vi "Create New File.vi"(8 "error in (no error)":errorcluster, 10 "Path":path, 11 "CSV File in":refnum<class "CSV File.lvclass">) -> (0 "error out":errorcluster, 1 "path out":path, 2 "File Refnum":variant, 3 "CSV File out":refnum<class "CSV File.lvclass">)   [LabVIEW 2021, in "CSV File.lvclass"]
doc: "This vi helps to create CSV file and output a file reference as a variant."
uses:
  CSV File.lvclass
  File Abstract Class/File Abstract.lvclass
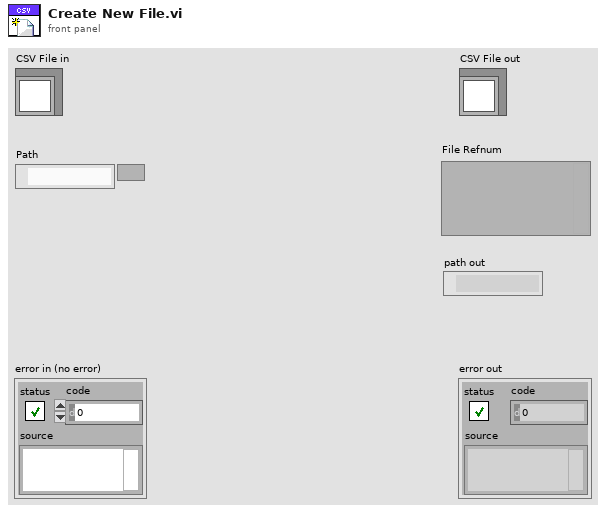
[diagram p1: front panel]
types:
  T1 = enum16{"open", "replace", "create", "open or create", "replace or create", "replace or create with confirmation"}
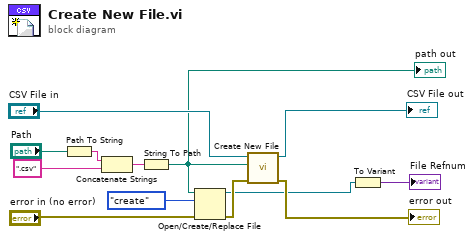
[diagram p0: block diagram]
diagram:
  n1 = Path To String(path="Path") -> (string=w4:string)
  n2 = Concatenate Strings(w4, ".csv") -> (w5:string)
  n3 = String To Path(string=w5) -> (path=w1:path)
  "path out" <- w1
  n4 = Open/Create/Replace File(file path (use dialog)=w1, error in="error in (no error)", operation (0:open)=T1."create") -> (refnum out=w7:refnum<file>, error out=w9:errorcluster)  [unwired: 3 in, 1 out]
  n5 = call-parent "Create New File.vi"("error in (no error)"=w9, "Path"=w1, "File Manager in"="CSV File in") -> ("error out"=→"error out":errorcluster, "File Manager out"=→"CSV File out":refnum<class "CSV File.lvclass">)  [unwired: 5 in, 2 out]
  n6 = To Variant(anything=w7) -> (Variant=→"File Refnum":variant)
